vi "progAspicSequence3.vi"(0 "PixelNumber":u32[](array[numeric])=[0] format="%07x", 2 "TriggerSelect":u32[](array[numeric])=[0] format="%07x") -> (9 "error out":errorcluster)   [LabVIEW 2014]
panel:
  out "PixelNumber 2":u32[](array[numeric]) format="%07x"
  in  "cabacmessagetype":u32=13107 format="%x"
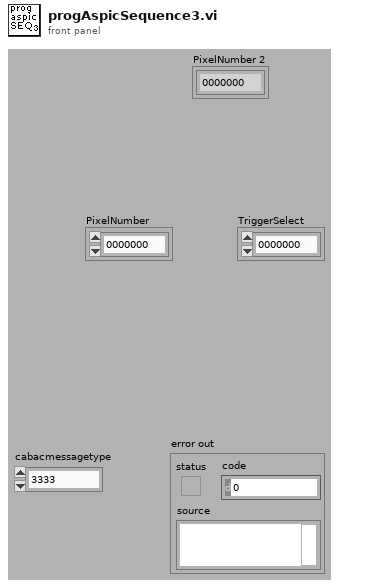
[diagram p1: front panel]
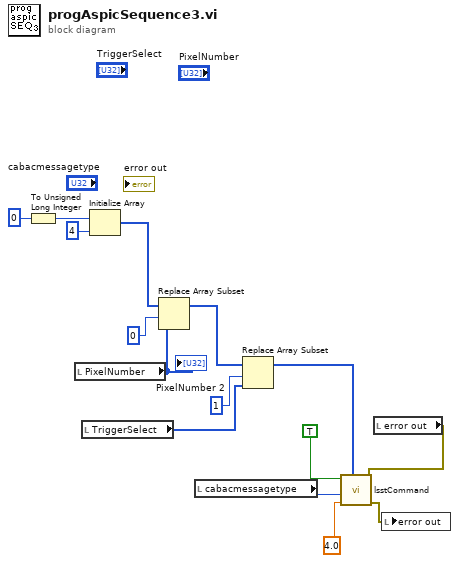
[diagram p0: block diagram]
diagram:
  n1 = To Unsigned Long Integer(number=u32 0 ("element")) -> (unsigned 32bit integer=w11:u32)
  n2 = local read "PixelNumber"() -> (w1:u32[])
  "PixelNumber 2" <- w1
  n3 = local read "TriggerSelect"() -> (w8:u32[])
  n4 = Initialize Array(w11, 4 ("dimension size")) -> (w3:u32[])
  n5 = Replace Array Subset(array=w3, new element=w1, index=0) -> (w2:u32[])
  n6 = local read "cabacmessagetype"() -> (w14:u32)
  n7 = Replace Array Subset(array=w2, new element=w8, index=1) -> (w7:u32[])
  n8 = local read "error out"() -> (w5:errorcluster)
  n9 = call "lsstCommand.vi"("error in (no error)"=w5, "data"=w7, "nbitems"=4.0, "messagetype"=w14, "execute"=TRUE) -> ("error out"=w15:errorcluster)  [unwired: 2 in, 4 out]
  n10 = local write "error out"(w15) -> ()
